vi "BRig_RT__Case_Exp__State_initTrial2__Laser_Wrong__v3.vi"(1 "input_L_OnOff":u16, 2 "input_L_Block":u16, 3 "input_L_Trial":u16, 4 "input_L_Probability":u16, 6 "input_nWrong":u16, 7 "input_nReward":u16, 8 "input_iSpout":u16, 9 "input_L_nRew1":u16, 10 "input_sState_start":u16, 11 "input_L_nRew2":u16, 12 "input_LaserSwitch":bool) -> (16 "output_LR_Event":bool, 17 "output_LR_Event_num":u16, 18 "output_LR_Laser":bool, 19 "output_LR_Laser_num":u16)   [LabVIEW 2014]
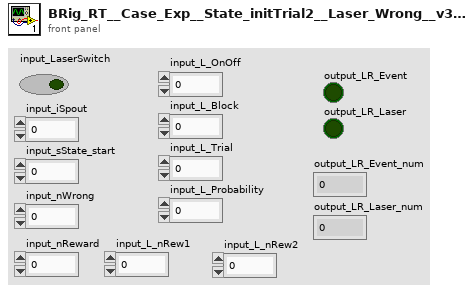
[diagram p1: front panel]
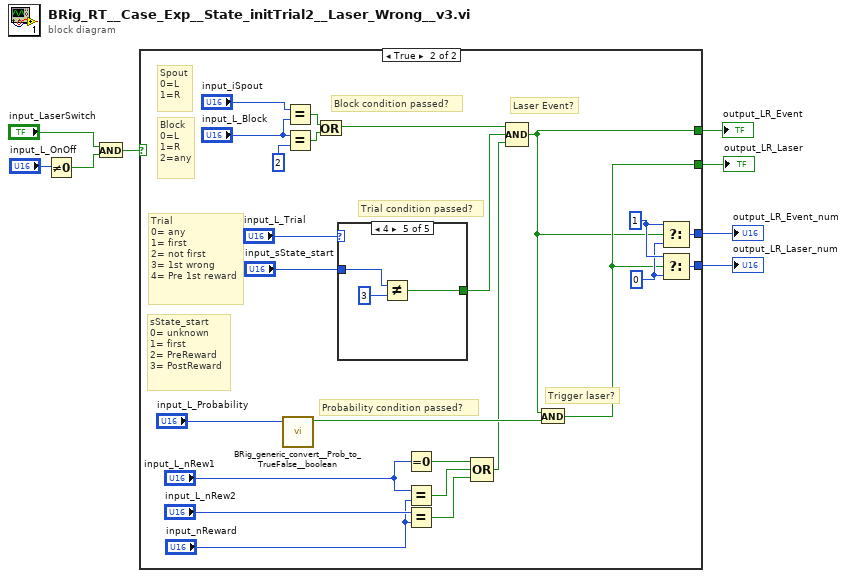
[diagram p0: block diagram]
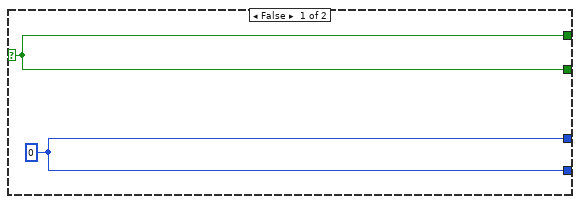
[diagram p2: hidden frame]
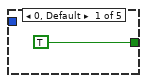
[diagram p3: hidden frame]
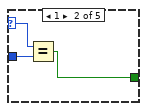
[diagram p4: hidden frame]
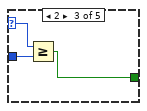
[diagram p5: hidden frame]
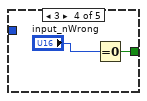
[diagram p6: hidden frame]
diagram:
  n1 = Not Equal To 0?(x="input_L_OnOff") -> (x != 0?=w7:bool)
  n2 = And(x="input_LaserSwitch", y=w7) -> (x .and. y?=w5:bool)
  n3 = case shown="True" w5 {
    selector: w5 -> [w10 _]
    tunnel: [w10 w20] -> w4
    tunnel: [w10 w21] -> w3
    tunnel: [w9 w19] -> w2
    tunnel: [w9 w18] -> w1
    frame False {
      w9 = u16 0 ("y")
    }
    frame True {
      w22 = u16 0 ("y")
      w23 = u16 1 ("y")
      # "Trigger laser?"
      # "Laser Event?"
      # "Trial condition passed?"
      # "sState_start\n0= unknown\n1= first\n2= PreReward\n3= PostReward"
      # "Probability condition passed?"
      # "Trial\n0= any\n1= first\n2= not first\n3= 1st wrong\n4= Pre 1st reward"
      # "Block condition passed?"
      # "Spout\n0=L\n1=R"
      # "Block\n0=L\n1=R\n2=any"
      n4 = call "BRig_generic_convert__Prob_to_TrueFalse__boolean.vi"("input_probability_u16"="input_L_Probability") -> ("output_TF"=w24:bool)  [unwired: 10 in]
      n5 = Equal?(x="input_iSpout", y="input_L_Block") -> (x = y?=w34:bool)
      n6 = Equal?(x="input_L_Block", y=u16 2) -> (x = y?=w33:bool)
      n7 = Or(x=w34, y=w33) -> (x .or. y?=w26:bool)
      n8 = case shown="4" "input_L_Trial" {
        selector: "input_L_Trial" -> [_ w37 w40 _ _]
        tunnel: [TRUE w36 w39 w43 w44] -> w25
        tunnel: "input_sState_start" -> [_ w38 w41 _ w46]
        frame 0, Default {
        }
        frame 1 {
          n9 = Equal?(x=w37, y=w38) -> (x = y?=w36:bool)
        }
        frame 2 {
          n10 = Greater Or Equal?(x=w40, y=w41) -> (x >= y?=w39:bool)
        }
        frame 3 {
          n11 = Equal To 0?(x="input_nWrong") -> (x = 0?=w43:bool)
        }
        frame 4 {
          n12 = Not Equal?(x=w46, y=u16 3) -> (x != y?=w44:bool)
        }
      }
      n13 = Equal To 0?(x="input_L_nRew1") -> (x = 0?=w17:bool)
      n14 = Equal?(x="input_L_nRew1", y="input_nReward") -> (x = y?=w16:bool)
      n15 = Equal?(x="input_L_nRew2", y="input_nReward") -> (x = y?=w15:bool)
      n16 = Compound Arithmetic op=OR(w17, w16, w15) -> (w12:bool)
      n17 = Compound Arithmetic op=AND(w26, w25, w12) -> (w20:bool)
      n18 = And(x=w20, y=w24) -> (x .and. y?=w21:bool)
      n19 = Select(t=w23, s=w20, f=w22) -> (s? t:f=w19:u16)
      n20 = Select(t=w23, s=w21, f=w22) -> (s? t:f=w18:u16)
    }
  }
  "output_LR_Event" <- w4
  "output_LR_Laser" <- w3
  "output_LR_Event_num" <- w2
  "output_LR_Laser_num" <- w1
